vi "Initialize.vi"(8 "error in (no error)":errorcluster, 9 "Channel":i32, 10 "VISA resource name":refnum<visa-resource-name>="COM9", 11 "YP03-60_Z in":refnum<class "YP03-60_Z.lvclass">) -> (0 "error out":errorcluster, 3 "YP03-60_Z out":refnum<class "YP03-60_Z.lvclass">)   [LabVIEW 2020, in "PowerControl.lvlib" / "YP03-60_Z.lvclass"]
uses:
  YP03-60_Z.lvclass
  VirtualPower/VirtualPower.lvclass
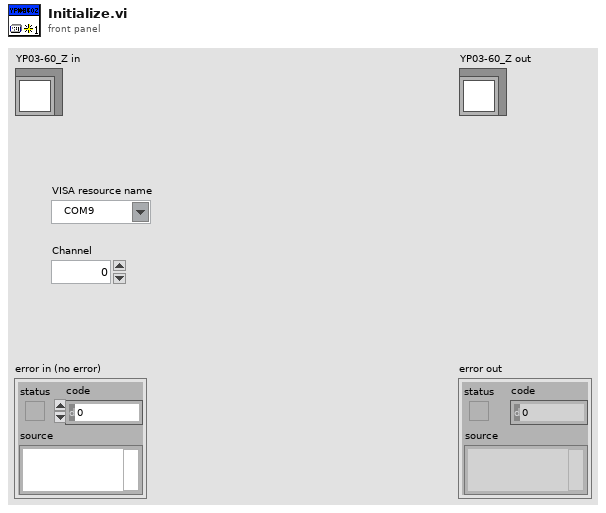
[diagram p1: front panel]
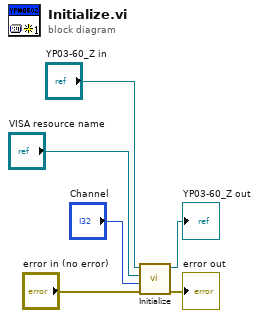
[diagram p0: block diagram]
diagram:
  n1 = call-parent "Initialize.vi"("error in (no error)"="error in (no error)", "Channel"="Channel", "VISA resource name"="VISA resource name", "VirtualPower in"="YP03-60_Z in") -> ("error out"=→"error out":errorcluster, "VirtualPower out"=→"YP03-60_Z out":refnum<class "YP03-60_Z.lvclass">)  [unwired: 6 in]
